vi "MissionOp Check Timeout.vi"(8 "error in (no error)":errorcluster, 11 "RDS Mission Controller Actor in":refnum<class "RDS Mission Controller Actor.lvclass">) -> (0 "error out":errorcluster, 3 "RDS Mission Controller Actor out":refnum<class "RDS Mission Controller Actor.lvclass">)   [LabVIEW 2015, in "RDS Mission Controller Actor.lvlib" / "RDS Mission Controller Actor.lvclass"]
uses:
  RDS Mission Controller Actor.lvclass
  RDS Mission Controller Actor.lvclass/RDS Mission Controller Actor.ctl
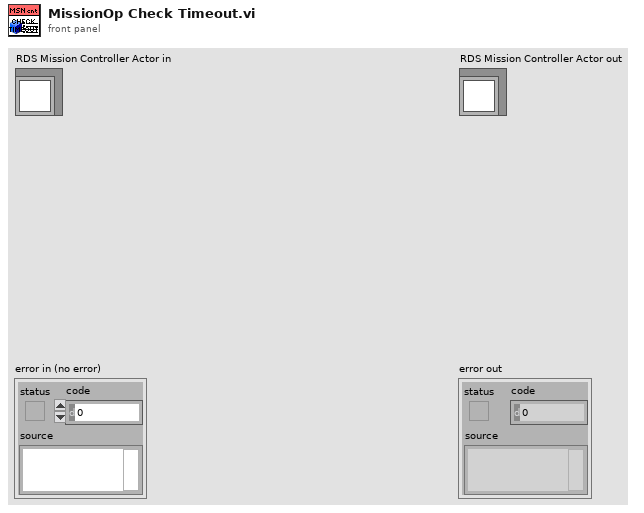
[diagram p1: front panel]
types:
  T1 = enum16{"Waypoint", "Loiter", "Wait", "Deploy AIP", "Stow AIP"}
  T2 = typedef "RDS Mission Controller Actor.lvlib/MissionOp.ctl" = cluster{"MissionOp Type":enum16{"Waypoint", "Loiter", "Wait", "Deploy AIP", "Stow AIP"}, "Duration (s)":u16, "Throttle":i16, "GPS Latitude":dbl, "GPS Longitude":dbl, "Loiter Range (m)":u16}
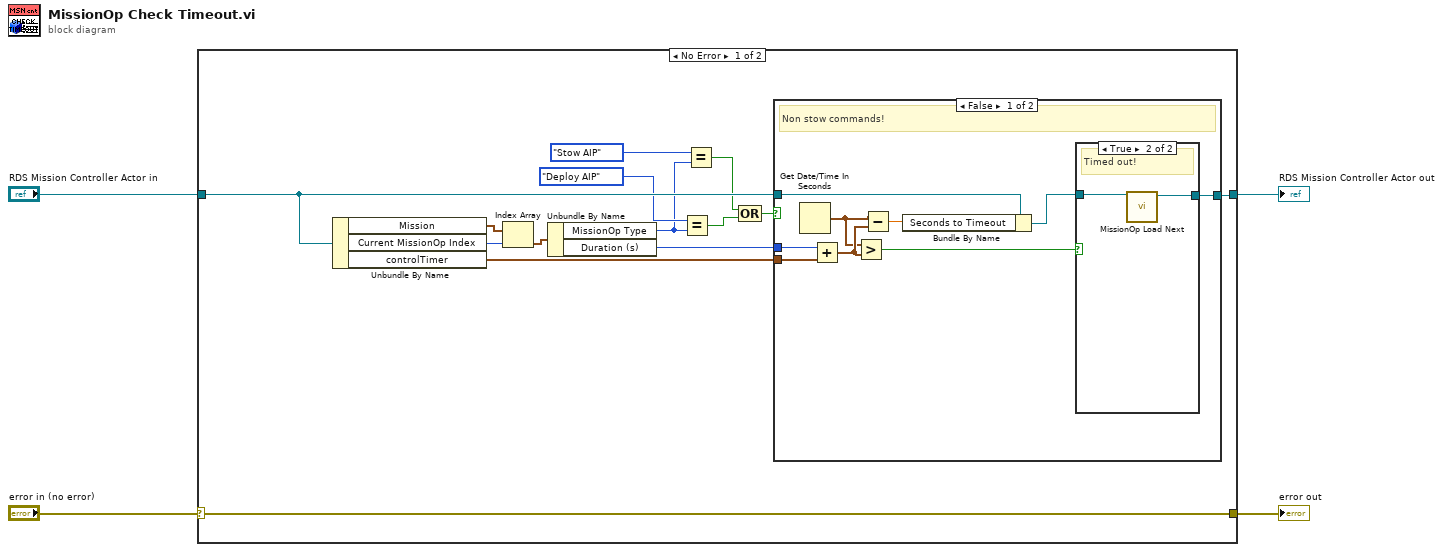
[diagram p0: block diagram]
diagram:
  n1 = case shown="No Error" "error in (no error)" {
    selector: "error in (no error)" -> [w18 w33]
    tunnel: [w18 w33] -> w3
    tunnel: [w13 w32] -> w1
    tunnel: "RDS Mission Controller Actor in" -> [w14 w32]
    frame No Error {
      n2 = Unbundle By Name(w14) -> ("Mission"=w17:T2[], "Current MissionOp Index"=w16:i32, "controlTimer"=w6:timestamp)
      n3 = Index Array(array=w17, index=w16) -> (element=w15:T2)
      n4 = Unbundle By Name(w15) -> ("MissionOp Type"=w8:T1, "Duration (s)"=w5:u16)
      n5 = Equal?(x=T1."Deploy AIP", y=w8) -> (x = y?=w10:bool)
      n6 = Equal?(x=T1."Stow AIP", y=w8) -> (x = y?=w7:bool)
      n7 = Compound Arithmetic op=OR(w7, w10) -> (w11:bool)
      n8 = case shown="False" w11 {
        tunnel: w5 -> [w27 _]
        tunnel: w6 -> [w26 _]
        tunnel: w14 -> [w20 w31]
        tunnel: [w24 w31] -> w13
        frame False {
          # "Non stow commands!"
          n9 = Get Date/Time In Seconds() -> (seconds since 1Jan1904=w22:timestamp)
          n10 = Add(x=w27, y=w26) -> (x+y=w23:timestamp)
          n11 = Greater?(x=w22, y=w23) -> (0:w25:bool)
          n12 = Subtract(x=w22, y=w23) -> (x-y=w21:dbl)
          n13 = Bundle By Name(cluster=w20, "Seconds to Timeout"=w21) -> (w19:refnum<class "RDS Mission Controller Actor.lvclass">)
          n14 = case shown="True" w25 {
            tunnel: w19 -> [w28 w30]
            tunnel: [w28 w29] -> w24
            frame False {
              # "Not timed out!"
            }
            frame True {
              # "Timed out!"
              n15 = call "MissionOp Load Next.vi"("RDS Mission Controller Actor in"=w30) -> ("RDS Mission Controller Actor out"=w29:refnum<class "RDS Mission Controller Actor.lvclass">)  [unwired: 9 in, 1 out]
            }
          }
        }
        frame True {
          # "Stow/deploy commands don't get timed out!"
        }
      }
    }
    frame Error {
    }
  }
  "error out" <- w3
  "RDS Mission Controller Actor out" <- w1
